vi "Create Transform from Translation.vi"(9 "z":dbl, 10 "y":dbl, 11 "x":dbl) -> (3 "transform":T1)   [LabVIEW 2017, in "NI_Kinematics.lvlib"]
doc: "Returns a homogenous transform that represents the translation of a point in one coordinate frame by values along the <B>x</B>-, <B>y</B>-, and <B>z</B>-axes to convert the point to coordinates of another coordinate frame."
uses:
  <vilib>/robotics/Kinematics/NI_Kinematics.lvlib
  <vilib>/Analysis/Matrix/Datatypes/RealMatrix.ctl
  <vilib>/Analysis/Matrix/NI_Matrix.lvlib
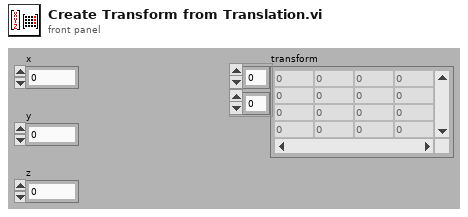
[diagram p1: front panel]
types:
  T1 = typedef "NI_Matrix.lvlib/RealMatrix.ctl" = dbl[][]
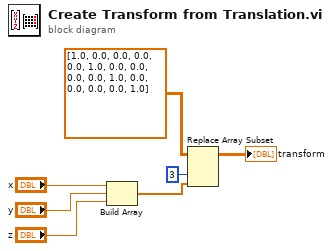
[diagram p0: block diagram]
diagram:
  n1 = Build Array("x", "y", "z") -> (w1:dbl[])
  n2 = Replace Array Subset(array=T1 [[1.0, 0.0, 0.0, 0.0], [0.0, 1.0, 0.0, 0.0], [0.0, 0.0, 1.0, 0.0], [0.0, 0.0, 0.0, 1.0]] ("A"), new element=w1, index (col)=3 ("disabled index (col)")) -> (→"transform":T1)  [unwired: 1 in]
